vi "Test - Draw Filled Triangle 1D.vi"() -> ()   [LabVIEW 2020, in "Raster (FPGA).lvlib"]
uses:
  Raster (FPGA).lvlib
  Rectangle Dimensions.ctl
  3D/Vector 3D.ctl
  3D/3D (FPGA).lvlib
  UV.ctl
  3D/Vertex.ctl
  3D/Triangle.ctl
panel:
  in  "Triangle":T1={"Vertex 1"={"Position"={"x"=75.0, "y"=25.0, "z"=0.0}, "UV"={"u"=0.0, "v"=0.0}, "Colour"=12517256}, "Vertex 2"={"Position"={"x"=500.0, "y"=450.0, "z"=0.0}, "UV"={"u"=0.0, "v"=0.0}, "Colour"=12517256}, "Vertex 3"={"Position"={"x"=50.0, "y"=200.0, "z"=0.0}, "UV"={"u"=0.0, "v"=0.0}, "Colour"=12517256}, "Colour"=0} {"Vertex 3"."UV"."v" min=0 max=1 step=0.1; "Vertex 3"."UV"."u" min=0 max=1 step=0.1; "Vertex 2"."UV"."v" min=0 max=1 step=0.1; "Vertex 2"."UV"."u" min=0 max=1 step=0.1; "Vertex 1"."UV"."v" min=0 max=1 step=0.1; "Vertex 1"."UV"."u" min=0 max=1 step=0.1}
  # "(0,0)"
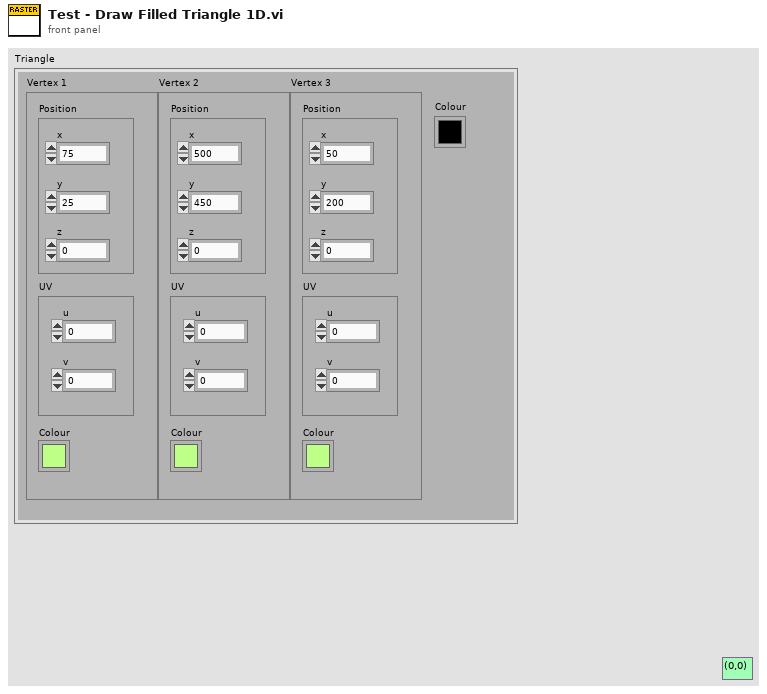
[diagram p1: front panel]
types:
  T1 = typedef "3D (FPGA).lvlib/Triangle.ctl" = cluster{"Vertex 1":T2, "Vertex 2":T2, "Vertex 3":T2, "Colour":u32}
  T2 = typedef "3D (FPGA).lvlib/Vertex.ctl" = cluster{"Position":T3, "UV":T4, "Colour":u32}
  T3 = typedef "3D (FPGA).lvlib/Vector 3D.ctl" = cluster{"x":sgl, "y":sgl, "z":sgl}
  T4 = typedef "Raster (FPGA).lvlib/UV.ctl" = cluster{"u":sgl, "v":sgl}
  T5 = typedef "Raster (FPGA).lvlib/Rectangle Dimensions.ctl" = cluster{"Width":u32, "Height":u32}
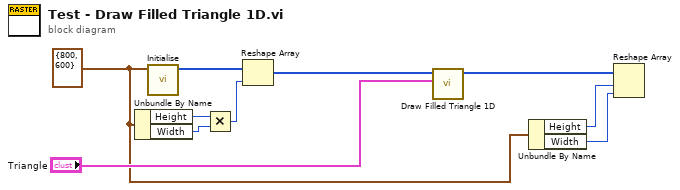
[diagram p0: block diagram]
diagram:
  w5 = T5 {"Width"=800, "Height"=600} ("Screen Dimensions")
  n1 = Unbundle By Name(w5) -> ("Height"=w8:u32, "Width"=w7:u32)
  n2 = call "Initialise.vi"("Screen Dimensions"=w5) -> ("Pixel Data out"=w9:u32[])  [unwired: 10 in]
  n3 = Multiply(x=w8, y=w7) -> (x*y=w6:u32)
  n4 = Reshape Array(w9, w6) -> (w2:u32[])
  n5 = call "Draw Filled Triangle 1D.vi"("Triangle"="Triangle", "Pixel Data in"=w2) -> ("Pixel Data out"=w1:u32[])  [unwired: 9 in]
  n6 = Unbundle By Name(w5) -> ("Height"=w4:u32, "Width"=w3:u32)
  n7 = Reshape Array(w1, w4, w3) -> ()  [unwired: 1 out]
